vi "Lookup.vi"(10 "Name":string, 11 "Variables in":refnum<class "Variables.lvclass">) -> (2 "error out":errorcluster, 3 "Index":i32)   [LabVIEW 2020, in "VolatusSeq.lvlib" / "Variables.lvclass"]
uses:
  Variables.lvclass
  Variables.lvclass/Variables.ctl
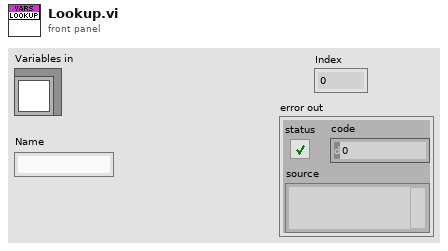
[diagram p1: front panel]
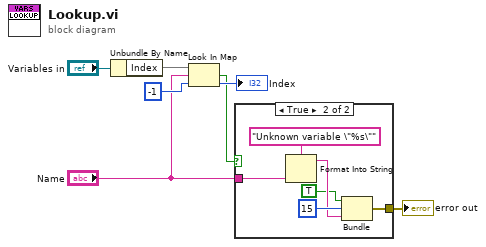
[diagram p0: block diagram]
diagram:
  n1 = Unbundle By Name("Variables in") -> ("Index"=w6:map{string, i32})
  n2 = Look In Map(map=w6, key="Name", default value=-1) -> (key not found?=w3:bool, value=→"Index":i32)
  n3 = case shown="True" w3 {
    tunnel: "Name" -> [_ w13]
    tunnel: [_ w8] -> w2
    frame False {
    }
    frame True {
      n4 = Format Into String(format string="Unknown variable \"%s\"", w13) -> (resulting string=w10:string)  [unwired: 2 in, 1 out]
      n5 = Bundle(TRUE, "Code"=15, w10) -> (w8:cluster{bool, "Code":i32, string})  [unwired: 1 in]
    }
  }
  "error out" <- w2
